vi "Error.vi"(11 "Dummy In":refnum<class "Example Test Case.lvclass">) -> (0 "error out":errorcluster, 3 "Dummy Out":refnum<class "Example Test Case.lvclass">)   [LabVIEW 2020, in "Example Test Case.lvclass"]
doc: "Test which fails due to an error"
uses:
  Example Test Case.lvclass
  C:/git/astemes-lunit/source/API/LUnit Test Case/LUnit Test Case.lvclass
  API/LUnit Test Case/LUnit Test Case.lvclass/LUnit Test Case.ctl
  API/LUnit Test Case/Private/Append Pass Result.vi
  API/LUnit Test Case/Private/Run In UI.vi
  <vilib>/Utility/error.llb/Clear Errors.vi
  Example Test Case.lvclass/Example Test Case.ctl
  API/LUnit Test Case/LUnit Test Case.lvclass
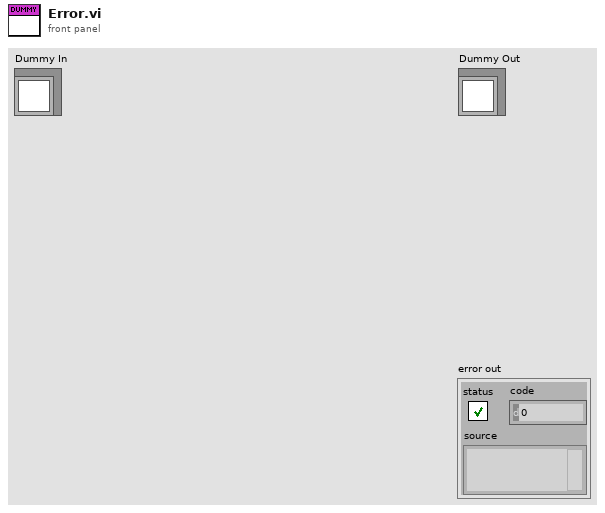
[diagram p1: front panel]
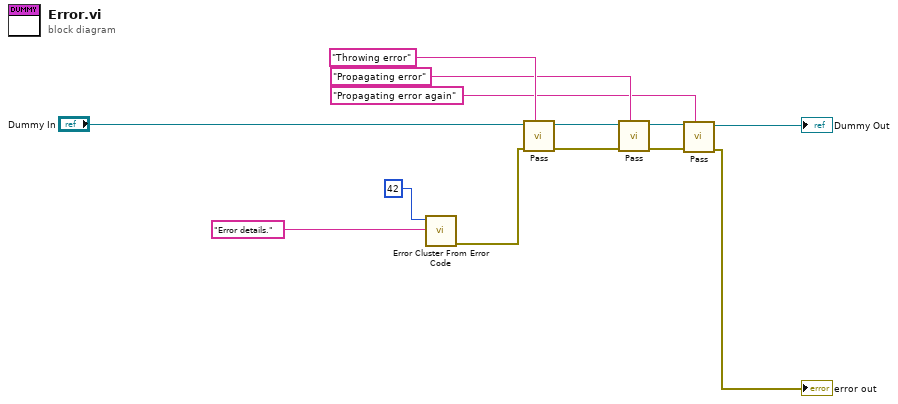
[diagram p0: block diagram]
diagram:
  n1 = call <vilib>:"Error Cluster From Error Code.vi"("error message (\"\")"="Error details." ("Description"), "error code (0)"=42) -> ("error out"=w9:errorcluster)  [unwired: 7 in]
  n2 = call "Pass.vi"("Description"="Throwing error", "error in (no error)"=w9, "LUnit Test Case In"="Dummy In") -> ("error out"=w7:errorcluster, "LUnit Test Case Out"=w5:refnum<class "Example Test Case.lvclass">)  [unwired: 7 in]
  n3 = call "Pass.vi"("Description"="Propagating error", "error in (no error)"=w7, "LUnit Test Case In"=w5) -> ("error out"=w8:errorcluster, "LUnit Test Case Out"=w4:refnum<class "Example Test Case.lvclass">)  [unwired: 7 in]
  n4 = call "Pass.vi"("Description"="Propagating error again", "error in (no error)"=w8, "LUnit Test Case In"=w4) -> ("error out"=→"error out":errorcluster, "LUnit Test Case Out"=→"Dummy Out":refnum<class "Example Test Case.lvclass">)  [unwired: 7 in]
